vi "Get 1 Algorithm Info.vi"(6 "Backend engine":T1, 8 "error in (no error)":errorcluster, 11 "Algorithm ID":string) -> (0 "error out":errorcluster, 3 "Algorithm Information":T2)   [LabVIEW 2013, in "QWTBLVLib.lvlib"]
doc: "Returns informations on one algorithm."
uses:
  QWTBLVLib.lvlib
  TD Algorithm Information.ctl
  TD Backend Engine.ctl
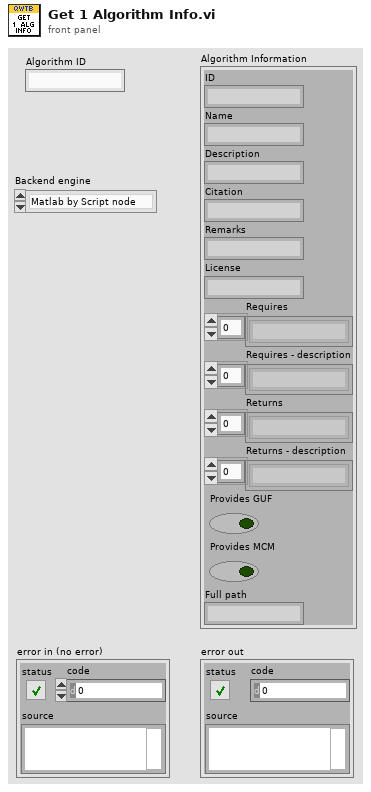
[diagram p1: front panel]
types:
  T1 = typedef "QWTBLVLib.lvlib/TD Backend Engine.ctl" = enum16{"Matlab by Script node", "GNU Octave by GOLPI"}
  T2 = typedef "QWTBLVLib.lvlib/TD Algorithm Information.ctl" = cluster{"ID":string, "Name":string, "Description":string, "Citation":string, "Remarks":string, "License":string, "Requires":string[], "Requires - description":string[], "Returns":string[], "Returns - description":string[], "Provides GUF":bool, "Provides MCM":bool, "Full path":string}
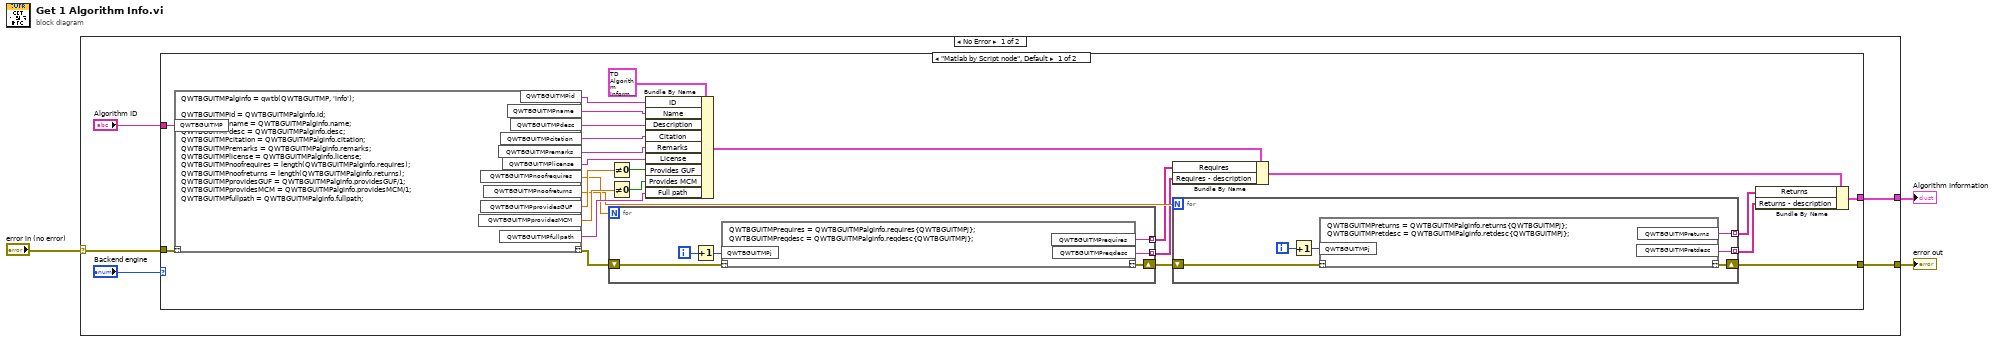
[diagram p0: block diagram]
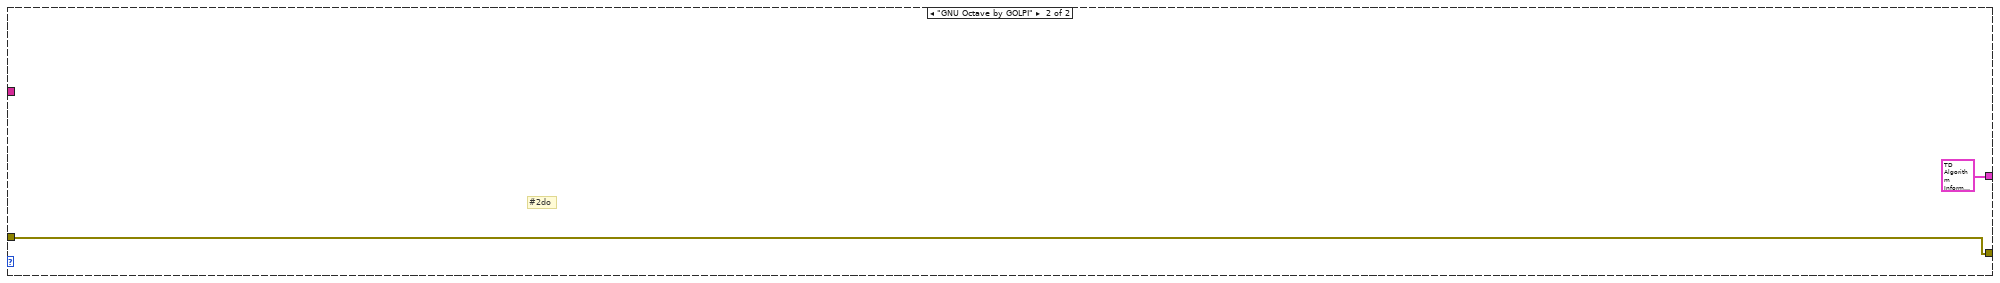
[diagram p2: hidden frame]
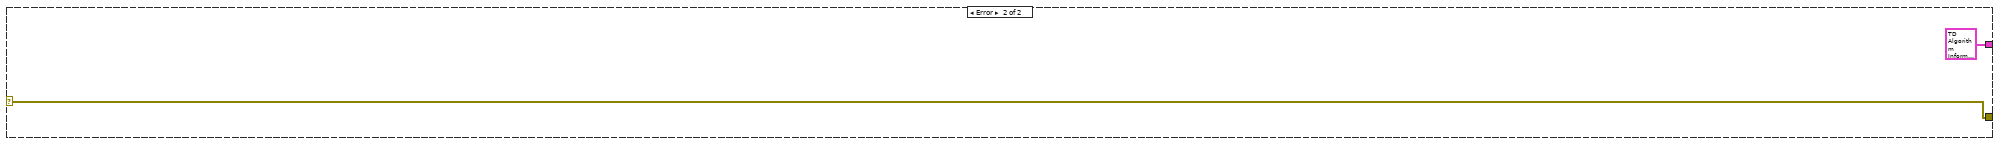
[diagram p3: hidden frame]
diagram:
  n1 = case shown="No Error" "error in (no error)" {
    selector: "error in (no error)" -> [w5 w49]
    tunnel: [w7 w49] -> w3
    tunnel: [w6 T2 {"ID"="", "Name"="", "Description"="", "Citation"="", "Remarks"="", "License"="", "Requires"=[], "Requires - description"=[], "Returns"=[], "Returns - description"=[], "Provides GUF"=FALSE, "Provides MCM"=FALSE, "Full path"=""} ("Algorithm Information")] -> w2
    frame No Error {
      n2 = case shown="\"Matlab by Script node\", Default" "Backend engine" {
        tunnel: "Algorithm ID" -> [w18 _]
        tunnel: [w11 w47] -> w7
        tunnel: [w10 T2 {"ID"="", "Name"="", "Description"="", "Citation"="", "Remarks"="", "License"="", "Requires"=[], "Requires - description"=[], "Returns"=[], "Returns - description"=[], "Provides GUF"=FALSE, "Provides MCM"=FALSE, "Full path"=""} ("Algorithm Information")] -> w6
        tunnel: w5 -> [w9 w47]
        frame "Matlab by Script node", Default {
          n3 = script code="QWTBGUITMPalginfo = qwtb(QWTBGUITMP, 'info');\n\nQWTBGUITMPid = QWTBGUITMPalginfo.id;\nQWTBGUITMPname = QWTBGUITMPalginfo.name;\nQWTBGUITMPdesc = QWTBGUITMPalginfo.desc;\nQWTBGUITMPcitation = QWTBGUITMPalginfo.citation;\nQWTBGUITMPremarks = QWTBGUITMPalginfo.remarks;\nQWTBGUITMPlicense = QWTBGUITMPalginfo.license;\nQWTBGUITMPnoofrequires = length(QWTBGUITMPalginfo.requires);\nQWTBGUITMPnoofreturns = length(QWTBGUITMPalginfo.returns);\nQWTBGUITMPprovidesGUF = QWTBGUITMPalginfo.providesGUF/1;\nQWTBGUITMPprovidesMCM = QWTBGUITMPalginfo.providesMCM/1;\nQWTBGUITMPfullpath = QWTBGUITMPalginfo.fullpath;"("??"=w9, "QWTBGUITMP"=w18) -> ("??"=w22:errorcluster, "QWTBGUITMPid"=w32:string, "QWTBGUITMPname"=w31:string, "QWTBGUITMPdesc"=w30:string, "QWTBGUITMPfullpath"=w29:string, "QWTBGUITMPnoofrequires"=w21:dbl, "QWTBGUITMPnoofreturns"=w19:dbl, "QWTBGUITMPcitation"=w23:string, "QWTBGUITMPremarks"=w24:string, "QWTBGUITMPprovidesGUF"=w26:dbl, "QWTBGUITMPprovidesMCM"=w28:dbl, "QWTBGUITMPlicense"=w34:string)
          n4 = for {
            N: w21 -> [_]
            shift-right: [w43] -> w20
            shift-left: w22 -> [w46]
            tunnel: [w42] -> w15 mode=indexing
            tunnel: [w41] -> w14 mode=indexing
            i -> [w44]
            n5 = Increment(x=w44) -> (x+1=w45:i32)
            n6 = script code="QWTBGUITMPrequires = QWTBGUITMPalginfo.requires{QWTBGUITMPj};\nQWTBGUITMPreqdesc = QWTBGUITMPalginfo.reqdesc{QWTBGUITMPj};"("??"=w46, "QWTBGUITMPj"=w45) -> ("??"=w43:errorcluster, "QWTBGUITMPrequires"=w42:string, "QWTBGUITMPreqdesc"=w41:string)
          }
          n7 = Not Equal To 0?(x=w26) -> (x != 0?=w25:bool)
          n8 = Not Equal To 0?(x=w28) -> (x != 0?=w27:bool)
          n9 = Bundle By Name(cluster=T2 {"ID"="", "Name"="", "Description"="", "Citation"="", "Remarks"="", "License"="", "Requires"=[], "Requires - description"=[], "Returns"=[], "Returns - description"=[], "Provides GUF"=FALSE, "Provides MCM"=FALSE, "Full path"=""} ("Algorithm Information"), "ID"=w32, "Name"=w31, "Description"=w30, "Citation"=w23, "Remarks"=w24, "License"=w34, "Provides GUF"=w25, "Provides MCM"=w27, "Full path"=w29) -> (w13:T2)
          n10 = Bundle By Name(cluster=w13, "Requires"=w15, "Requires - description"=w14) -> (w12:T2)
          n11 = for {
            N: w19 -> [_]
            shift-right: [w37] -> w11
            shift-left: w20 -> [w40]
            tunnel: [w36] -> w16 mode=indexing
            tunnel: [w35] -> w17 mode=indexing
            i -> [w38]
            n12 = Increment(x=w38) -> (x+1=w39:i32)
            n13 = script code="QWTBGUITMPreturns = QWTBGUITMPalginfo.returns{QWTBGUITMPj};\nQWTBGUITMPretdesc = QWTBGUITMPalginfo.retdesc{QWTBGUITMPj};"("??"=w40, "QWTBGUITMPj"=w39) -> ("??"=w37:errorcluster, "QWTBGUITMPreturns"=w36:string, "QWTBGUITMPretdesc"=w35:string)
          }
          n14 = Bundle By Name(cluster=w12, "Returns"=w16, "Returns - description"=w17) -> (w10:T2)
        }
        frame "GNU Octave by GOLPI" {
          # "#2do"
        }
      }
    }
    frame Error {
    }
  }
  "error out" <- w3
  "Algorithm Information" <- w2
